vi "points to mm.vi"(3 "points":sgl) -> (0 "mm":sgl)   [LabVIEW 2019]
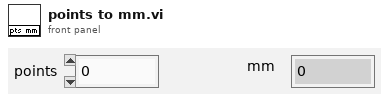
[diagram p1: front panel]
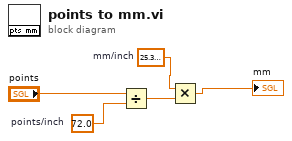
[diagram p0: block diagram]
diagram:
  w2 = sgl 25.4  # mm/inch
  w3 = sgl 72.0  # points/inch
  n1 = Divide(x="points", y=w3) -> (x/y=w5:sgl)
  n2 = Multiply(x=w2, y=w5) -> (x*y=→"mm":sgl)
